vi "Persistence Test.vi"() -> (0 "error out":errorcluster)   [LabVIEW 2014, in "SQLite3LV Tests.lvlib"]
uses:
  SQLite3LV Tests.lvlib
  SQLite3LV/SQLite3 Class/struct_table_info.ctl
  SQLite3LV/SQLite3 Class/sqlite3.lvclass
  SQLite3LV/Cursor Class/cursor.lvclass
  SQLite3LV/SQLite3LV.lvlib
panel:
  out "table info.":T1[](array[typedef])
  out "exists? 2":bool
  out "exists?":bool
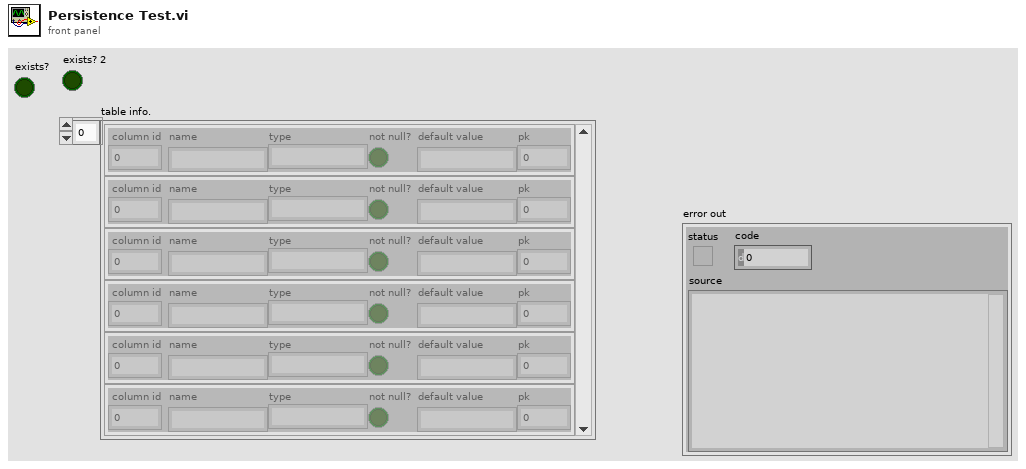
[diagram p1: front panel]
types:
  T1 = typedef "SQLite3LV.lvlib/struct_table_info.ctl" = cluster{" column id":i32, "name":string, "type":string, "not null?":bool, "default value":string, "pk":i32}
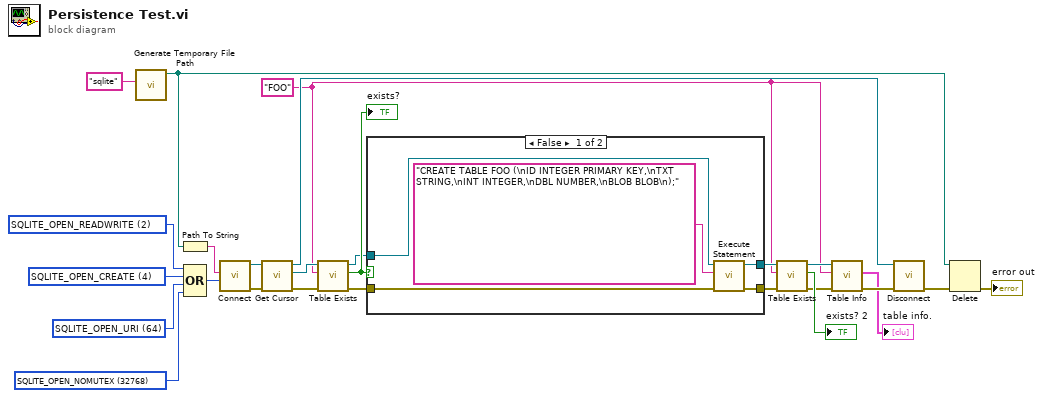
[diagram p0: block diagram]
diagram:
  w4 = "FOO" ("table")
  w24 = u32 32768 items=["SQLITE_OPEN_READONLY"=1, "SQLITE_OPEN_READWRITE"=2, "SQLITE_OPEN_CREATE"=4, "SQLITE_OPEN_DELETEONCLOSE"=8, "SQLITE_OPEN_EXCLUSIVE"=16, "SQLITE_OPEN_AUTOPROXY"=32, "SQLITE_OPEN_URI"=64, "SQLITE_OPEN_MEMORY"=128, "SQLITE_OPEN_MAIN_DB"=256, "SQLITE_OPEN_TEMP_DB"=512, "SQLITE_OPEN_TRANSIENT_DB"=1024, "SQLITE_OPEN_MAIN_JOURNAL"=2048, "SQLITE_OPEN_TEMP_JOURNAL"=4096, "SQLITE_OPEN_SUBJOURNAL"=8192, "SQLITE_OPEN_MASTER_JOURNAL"=16384, "SQLITE_OPEN_NOMUTEX"=32768, "SQLITE_OPEN_FULLMUTEX"=65536, "SQLITE_OPEN_SHAREDCACHE"=131072, "SQLITE_OPEN_PRIVATECACHE"=262144, "SQLITE_OPEN_WAL"=524288] ("SQLITE3 Open Flag")
  w23 = u32 64 items=["SQLITE_OPEN_READONLY"=1, "SQLITE_OPEN_READWRITE"=2, "SQLITE_OPEN_CREATE"=4, "SQLITE_OPEN_DELETEONCLOSE"=8, "SQLITE_OPEN_EXCLUSIVE"=16, "SQLITE_OPEN_AUTOPROXY"=32, "SQLITE_OPEN_URI"=64, "SQLITE_OPEN_MEMORY"=128, "SQLITE_OPEN_MAIN_DB"=256, "SQLITE_OPEN_TEMP_DB"=512, "SQLITE_OPEN_TRANSIENT_DB"=1024, "SQLITE_OPEN_MAIN_JOURNAL"=2048, "SQLITE_OPEN_TEMP_JOURNAL"=4096, "SQLITE_OPEN_SUBJOURNAL"=8192, "SQLITE_OPEN_MASTER_JOURNAL"=16384, "SQLITE_OPEN_NOMUTEX"=32768, "SQLITE_OPEN_FULLMUTEX"=65536, "SQLITE_OPEN_SHAREDCACHE"=131072, "SQLITE_OPEN_PRIVATECACHE"=262144, "SQLITE_OPEN_WAL"=524288] ("SQLITE3 Open Flag")
  w25 = u32 4 items=["SQLITE_OPEN_READONLY"=1, "SQLITE_OPEN_READWRITE"=2, "SQLITE_OPEN_CREATE"=4, "SQLITE_OPEN_DELETEONCLOSE"=8, "SQLITE_OPEN_EXCLUSIVE"=16, "SQLITE_OPEN_AUTOPROXY"=32, "SQLITE_OPEN_URI"=64, "SQLITE_OPEN_MEMORY"=128, "SQLITE_OPEN_MAIN_DB"=256, "SQLITE_OPEN_TEMP_DB"=512, "SQLITE_OPEN_TRANSIENT_DB"=1024, "SQLITE_OPEN_MAIN_JOURNAL"=2048, "SQLITE_OPEN_TEMP_JOURNAL"=4096, "SQLITE_OPEN_SUBJOURNAL"=8192, "SQLITE_OPEN_MASTER_JOURNAL"=16384, "SQLITE_OPEN_NOMUTEX"=32768, "SQLITE_OPEN_FULLMUTEX"=65536, "SQLITE_OPEN_SHAREDCACHE"=131072, "SQLITE_OPEN_PRIVATECACHE"=262144, "SQLITE_OPEN_WAL"=524288] ("SQLITE3 Open Flag")
  w26 = u32 2 items=["SQLITE_OPEN_READONLY"=1, "SQLITE_OPEN_READWRITE"=2, "SQLITE_OPEN_CREATE"=4, "SQLITE_OPEN_DELETEONCLOSE"=8, "SQLITE_OPEN_EXCLUSIVE"=16, "SQLITE_OPEN_AUTOPROXY"=32, "SQLITE_OPEN_URI"=64, "SQLITE_OPEN_MEMORY"=128, "SQLITE_OPEN_MAIN_DB"=256, "SQLITE_OPEN_TEMP_DB"=512, "SQLITE_OPEN_TRANSIENT_DB"=1024, "SQLITE_OPEN_MAIN_JOURNAL"=2048, "SQLITE_OPEN_TEMP_JOURNAL"=4096, "SQLITE_OPEN_SUBJOURNAL"=8192, "SQLITE_OPEN_MASTER_JOURNAL"=16384, "SQLITE_OPEN_NOMUTEX"=32768, "SQLITE_OPEN_FULLMUTEX"=65536, "SQLITE_OPEN_SHAREDCACHE"=131072, "SQLITE_OPEN_PRIVATECACHE"=262144, "SQLITE_OPEN_WAL"=524288] ("SQLITE3 Open Flag")
  n1 = call <vilib>:"Generate Temporary File Path.vi"("Temporary File Extension (tmp)"="sqlite") -> ("Unique Temporary File Path"=w20:path)  [unwired: 9 in, 1 out]
  n2 = Path To String(path=w20) -> (string=w19:string)
  n3 = Compound Arithmetic op=OR(w26, w25, w23, w24) -> (w18:u32)
  n4 = call "Connect.vi"("SQLITE3 open flags"=w18, "path"=w19) -> ("error out"=w16:errorcluster, "SQLite3LV Connection out"=w17:refnum<class "sqlite3.lvclass">)  [unwired: 8 in]
  n5 = call "Get Cursor.vi"("error in (no error)"=w16, "SQLite3LV Connection in"=w17) -> ("error out"=w13:errorcluster, "SQLite3LV Cursor"=w14:refnum<class "cursor.lvclass">, "SQLite3LV Connection out"=w15:refnum<class "sqlite3.lvclass">)  [unwired: 7 in]
  n6 = call "Table Exists.vi"("error in (no error)"=w13, "table"=w4, "SQLite3LV Cursor in"=w14) -> ("error out"=w10:errorcluster, "exists?"=w12:bool, "SQLite3LV Cursor out"=w11:refnum<class "cursor.lvclass">)  [unwired: 6 in]
  "exists?" <- w12
  n7 = case shown="False" w12 {
    tunnel: w11 -> [w31 w32]
    tunnel: w10 -> [w29 w33]
    tunnel: [w28 w33] -> w9
    tunnel: [w27 w32] -> w8
    frame False {
      n8 = call "Execute Statement.vi"("error in (no error)"=w29, "SQL statement"="CREATE TABLE FOO (\nID INTEGER PRIMARY KEY,\nTXT STRING,\nINT INTEGER,\nDBL NUMBER,\nBLOB BLOB\n);" ("statement"), "SQLite3LV Cursor in"=w31) -> ("error out"=w28:errorcluster, "SQLite3LV Cursor out"=w27:refnum<class "cursor.lvclass">)  [unwired: 7 in]
    }
    frame True {
    }
  }
  n9 = call "Table Exists.vi"("error in (no error)"=w9, "table"=w4, "SQLite3LV Cursor in"=w8) -> ("error out"=w5:errorcluster, "exists?"=→"exists? 2":bool, "SQLite3LV Cursor out"=w6:refnum<class "cursor.lvclass">)  [unwired: 6 in]
  n10 = call "Table Info.vi"("error in (no error)"=w5, "table"=w4, "SQLite3LV Cursor in"=w6) -> ("error out"=w3:errorcluster, "table info."=→"table info.":T1[])  [unwired: 6 in, 1 out]
  n11 = call "Disconnect.vi"("error in (no error)"=w3, "SQLite3LV Connection in"=w15) -> ("error out"=w1:errorcluster)  [unwired: 9 in]
  n12 = Delete(path (use dialog)=w20, error in=w1) -> (error out=→"error out":errorcluster)  [unwired: 3 in, 2 out]
